vi "AddToTopicsGlobal.vi"(3 "ROS in":T1) -> (1 "ROS out":T1)   [LabVIEW 2016]
doc: "Adds a topic to the global topic list"
uses:
  _ROSControl.ctl
  _ROSDirection.ctl
  _ROSDefinition.vi
panel:
  out "new?":bool
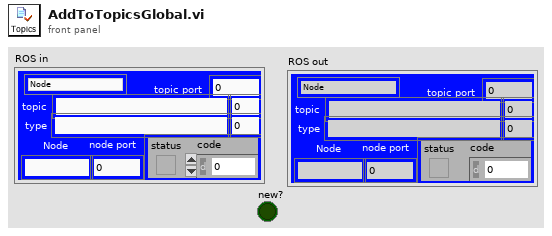
[diagram p1: front panel]
types:
  T1 = typedef "_ROSControl.ctl" = cluster{"topic port":u16, "Node":string, "topic":string, "type":string, "node port":u16, "error ":errorcluster, "Direction":T2, "Update (ms)":u16, "FIFO size":u16}
  T2 = typedef "_ROSDirection.ctl" = enum16{"Node", "Publisher", "Subscriber", "ServiceClient", "ServiceProvider"}
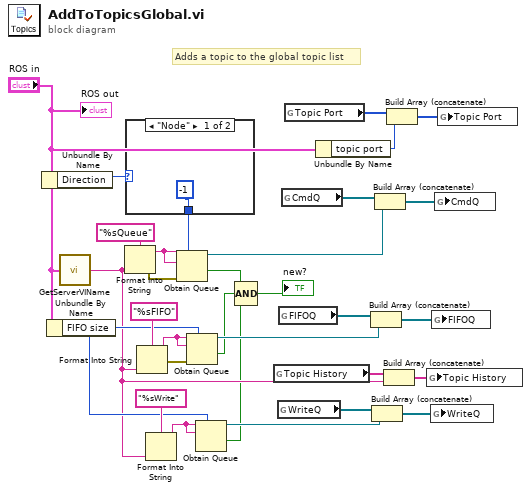
[diagram p0: block diagram]
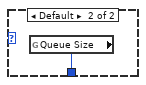
[diagram p2: hidden frame]
diagram:
  # "Adds a topic to the global topic list"
  n1 = Unbundle By Name("ROS in") -> ("Direction"=w9:T2)
  n2 = Unbundle By Name("ROS in") -> ("FIFO size"=w4:u16)
  n3 = call "GetServerVIName.vi"("ROS"="ROS in") -> ("vi name"=w3:string)
  n4 = Format Into String(format string="%sQueue" ("name (unnamed)"), w3) -> (resulting string=w29:string, error out=w30:errorcluster)  [unwired: 2 in]
  n5 = case shown="\"Node\"" w9 {
    tunnel: [-1 ("Queue Size") w33] -> w31
    frame "Node" {
    }
    frame Default {
      n6 = global read "_ROSDefinition.vi" "Queue Size"() -> (w33:i32)
    }
  }
  n7 = Format Into String(format string="%sFIFO" ("name (unnamed)"), w3) -> (resulting string=w25:string, error out=w26:errorcluster)  [unwired: 2 in]
  n8 = Format Into String(format string="%sWrite" ("name (unnamed)"), w3) -> (resulting string=w6:string)  [unwired: 2 in, 1 out]
  n9 = Obtain Queue(max queue size (-1, unlimited)=w31, name (unnamed)=w29, element data type=w29, error in (no error)=w30) -> (queue out=w24:refnum<queue>, created new?=w13:bool)  [unwired: 1 in, 1 out]
  n10 = Obtain Queue(max queue size (-1, unlimited)=w4, name (unnamed)=w25, element data type=w25, error in (no error)=w26) -> (queue out=w23:refnum<queue>, created new?=w12:bool)  [unwired: 1 in, 1 out]
  n11 = Obtain Queue(max queue size (-1, unlimited)=w4, name (unnamed)=w6, element data type=w6) -> (queue out=w2:refnum<queue>, created new?=w1:bool)  [unwired: 2 in, 1 out]
  n12 = Compound Arithmetic op=AND(w13, w12, w1) -> (→"new?":bool)
  n13 = global read "_ROSDefinition.vi" "Topic History"() -> (w22:string[])
  n14 = global read "_ROSDefinition.vi" "WriteQ"() -> (w8:refnum<queue>[])
  n15 = global read "_ROSDefinition.vi" "FIFOQ"() -> (w14:refnum<queue>[])
  n16 = global read "_ROSDefinition.vi" "CmdQ"() -> (w17:refnum<queue>[])
  n17 = global read "_ROSDefinition.vi" "Topic Port"() -> (w19:u16[])
  n18 = Unbundle By Name("ROS in") -> ("topic port"=w18:u16)
  n19 = Build Array (concatenate)(w14, w23) -> (w15:refnum<queue>[])
  n20 = Build Array (concatenate)(w8, w2) -> (w7:refnum<queue>[])
  n21 = Build Array (concatenate)(w17, w24) -> (w16:refnum<queue>[])
  n22 = Build Array (concatenate)(w22, w3) -> (w21:string[])
  n23 = Build Array (concatenate)(w19, w18) -> (w20:u16[])
  n24 = global write "_ROSDefinition.vi" "Topic History"(w21) -> ()
  n25 = global write "_ROSDefinition.vi" "WriteQ"(w7) -> ()
  n26 = global write "_ROSDefinition.vi" "FIFOQ"(w15) -> ()
  n27 = global write "_ROSDefinition.vi" "CmdQ"(w16) -> ()
  n28 = global write "_ROSDefinition.vi" "Topic Port"(w20) -> ()
  "ROS out" <- "ROS in"
